vi "Agilent VNA Set Stimulus.vi"(7 "Agilent VNA":T4={"Model"="8753C", "Serial"="", "Firmware"="", "Learn String"=""}, 8 "error in (no error)":errorcluster, 9 "Channel":i8=1 min=1 max=99 step=1, 10 "Stimulus":T1={"Use Instrument Settings"=FALSE, "Blank Frequencies"=FALSE, "Sweep Type"=enum."Linear", "Sweep"={"Fstart"=500.0, "Fstop"=1500.0, "Units"=enum."MHz", "Points"=201}, "Power (dBm)"=999.0, "IFBW (Hz)"=-1.0, "Sweep Time (s)"=-1.0, "Calibration"={"State"=FALSE, "String"=""}} {"Sweep Time (s)" format="%.3g"}, 11 "VISA Resource Name":refnum<visa-resource-name>) -> (0 "error out":errorcluster {"code" format="%.0x"}, 3 "dup VISA Resource Name":refnum<visa-resource-name>)   [LabVIEW 2011]
uses:
  TypeDefs/Agilent VNA Instrument Info.ctl
  tests/S Parameter/TypeDefs/SP Stimulus Parameters.ctl
  tests/S Parameter/TypeDefs/SP Frequency Units.ctl
  tests/S Parameter/TypeDefs/SP Calibration State.ctl
  TypeDefs/Agilent VNA Sweep Type.ctl
  TypeDefs/Agilent VNA Trigger Mode.ctl
panel:
  in  "Case Constant\n(See Context Help)":bool
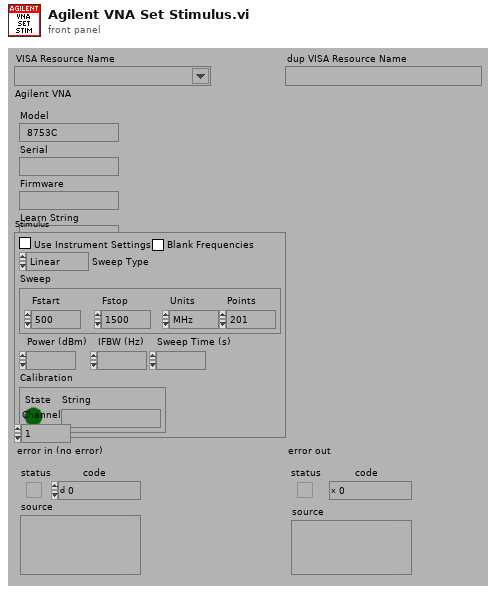
[diagram p1: front panel]
types:
  T1 = typedef "SP Stimulus Parameters.ctl" = cluster{"Use Instrument Settings":bool, "Blank Frequencies":bool, "Sweep Type":enum32{"Linear", "Logarithmic", "List", "Power", "CW"}, "Sweep":cluster{"Fstart":dbl, "Fstop":dbl, "Units":T2, "Points":i32}, "Power (dBm)":dbl, "IFBW (Hz)":dbl, "Sweep Time (s)":dbl, "Calibration":T3}
  T2 = typedef "SP Frequency Units.ctl" = enum16{"Hz", "kHz", "MHz", "GHz", "Points"}
  T3 = typedef "SP Calibration State.ctl" = cluster{"State":bool, "String":string}
  T4 = typedef "Agilent VNA Instrument Info.ctl" = cluster{"Model":string, "Serial":string, "Firmware":string, "Learn String":string}
  T5 = typedef "Agilent VNA Sweep Type.ctl" = enum32{"Linear Sweep", "Logarithmic Sweep", "Frequency List", "CW Time Sweep", "Power Sweep"}
  T6 = typedef "Agilent VNA Model.ctl" = enum16{"Not Supported", "8510X", "8719X", "8720X", "8722X", "8753X", "ENA", "PNA", "Field Fox"}
  T7 = typedef "Agilent VNA Trigger Mode.ctl" = enum16{"Continuous", "Hold", "Single"}
  T8 = enum32{"Linear", "Logarithmic", "List", "Power", "CW"}
  T9 = cluster{"Converted Frequency":dbl, "Converted Frequency":dbl}
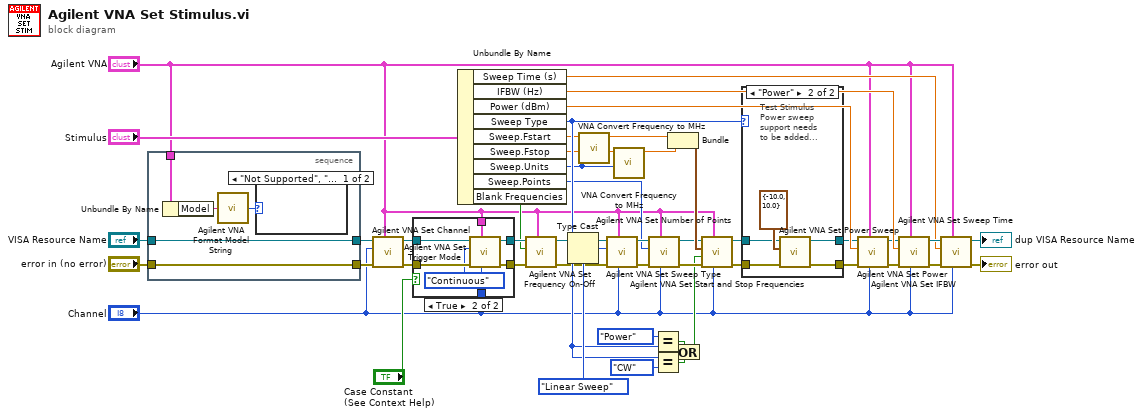
[diagram p0: block diagram]
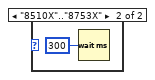
[diagram p3: hidden frame]
diagram:
  n1 = stacked-sequence {
    tunnel: "error in (no error)" -> [w52]
    tunnel: [w52] -> w34
    tunnel: "VISA Resource Name" -> [w51]
    tunnel: [w51] -> w32
    tunnel: "Agilent VNA" -> [w49]
    frame #0 {
      n2 = Unbundle By Name(w49) -> ("Model"=w48:string)
      n3 = call "Agilent VNA Format Model String.vi"("Model"=w48) -> ("Model"=w50:T6)
      n4 = case shown="\"Not Supported\", \"ENA\"..\"Field Fox\"" w50 {
        frame "Not Supported", "ENA".."Field Fox" {
        }
        frame "8510X".."8753X" {
          n5 = Wait (ms)(milliseconds to wait=u32 300) -> ()  [unwired: 1 out]
        }
      }
    }
  }
  n6 = call "Agilent VNA Set Channel.vi"("Agilent VNA"="Agilent VNA", "error in (no error)"=w34, "Channel"="Channel", "VISA Resource Name"=w32) -> ("error out"=w37:errorcluster, "dup VISA Resource Name"=w36:refnum<visa-resource-name>)  [unwired: 6 out]
  n7 = case shown="True" "Case Constant\n(See Context Help)" {
    tunnel: [w55 w59] -> w13
    tunnel: [w54 w60] -> w12
    tunnel: w37 -> [w55 w62]
    tunnel: w36 -> [w54 w61]
    tunnel: "Agilent VNA" -> [_ w57]
    tunnel: "Channel" -> [_ w56]
    frame False {
    }
    frame True {
      n8 = call "Agilent VNA Set Trigger Mode.vi"("Channel"=w56, "Agilent VNA"=w57, "error in (no error)"=w62, "Trigger Mode"=Agilent_VNA_Trigger_Mode."Continuous", "VISA Resource Name"=w61) -> ("error out"=w59:errorcluster, "dup VISA Resource Name"=w60:refnum<visa-resource-name>)  [unwired: 5 out]
    }
  }
  n9 = Unbundle By Name("Stimulus") -> ("Sweep Time (s)"=w40:dbl, "IFBW (Hz)"=w45:dbl, "Power (dBm)"=w46:dbl, "Sweep Type"=w16:T8, "Sweep.Fstart"=w6:dbl, "Sweep.Fstop"=w5:dbl, "Sweep.Units"=w4:T2, "Sweep.Points"=w7:i32, "Blank Frequencies"=w9:bool)
  n10 = call "Agilent VNA Set Frequency On-Off.vi"("Agilent VNA"="Agilent VNA", "error in (no error)"=w13, "Blank Frequencies (F)"=w9, "VISA Resource Name"=w12) -> ("error out"=w10:errorcluster, "dup VISA Resource Name"=w11:refnum<visa-resource-name>)  [unwired: 6 out]
  n11 = Type Cast(type=Agilent_VNA_Sweep_Type."Linear Sweep" ("Sweep Type"), x=w16) -> (*(type *) &x=w28:T5)
  n12 = call "VNA Convert Frequency to MHz.vi"("Units"=w4, "Frequency"=w6) -> ("Converted Frequency"=w3:dbl)  [unwired: 9 out]
  n13 = call "Agilent VNA Set Sweep Type.vi"("Channel"="Channel", "Agilent VNA"="Agilent VNA", "error in (no error)"=w10, "Sweep Type"=w28, "VISA Resource Name"=w11) -> ("error out"=w23:errorcluster, "dup VISA Resource Name"=w24:refnum<visa-resource-name>)  [unwired: 5 out]
  n14 = call "VNA Convert Frequency to MHz.vi"("Units"=w4, "Frequency"=w5) -> ("Converted Frequency"=w2:dbl)  [unwired: 9 out]
  n15 = call "Agilent VNA Set Number of Points.vi"("Channel"="Channel", "Agilent VNA"="Agilent VNA", "error in (no error)"=w23, "Number Points"=w7, "VISA Resource Name"=w24) -> ("error out"=w25:errorcluster, "dup VISA Resource Name"=w26:refnum<visa-resource-name>)  [unwired: 5 out]
  n16 = Equal?(x=enum32{"Linear", "Log", "List", "Power", "CW"}."Power" ("Sweep Type"), y=w16) -> (x = y?=w20:bool)
  n17 = Equal?(x=w16, y=enum32{"Linear", "Log", "List", "Power", "CW"}."CW" ("Sweep Type")) -> (x = y?=w19:bool)
  n18 = Bundle("Converted Frequency"=w3, "Converted Frequency"=w2) -> (w27:T9)  [unwired: 1 out]
  n19 = Or(x=w20, y=w19) -> (x .or. y?=w15:bool)
  n20 = call "Agilent VNA Set Start and Stop Frequencies.vi"("Channel"="Channel", "Agilent VNA"="Agilent VNA", "error in (no error)"=w25, "CW? (f)"=w15, "Start/Stop Freqs, MHz"=w27, "VISA Resource Name"=w26) -> ("error out"=w22:errorcluster, "dup VISA Resource Name"=w21:refnum<visa-resource-name>)  [unwired: 4 out]
  n21 = case shown="\"Power\"" w16 {
    tunnel: w22 -> [w64 w66]
    tunnel: w21 -> [w63 w65]
    tunnel: [w63 w68] -> w44
    tunnel: [w64 w67] -> w43
    frame "Linear", "Logarithmic", "CW", Default {
    }
    frame "Power" {
      # "Test Stimulus\nPower sweep\nsupport needs\nto be added..."
      n22 = call "Agilent VNA Set Power Sweep.vi"("error in (no error)"=w66, "Start/Stop Power, dBm"=cluster{"Pstart":dbl, "Pstop":dbl} {"Pstart"=-10.0, "Pstop"=10.0}, "VISA Resource Name"=w65) -> ("error out"=w67:errorcluster, "dup VISA Resource Name"=w68:refnum<visa-resource-name>)  [unwired: 7 out]
    }
  }
  n23 = call "Agilent VNA Set Power.vi"("Channel"="Channel", "Agilent VNA"="Agilent VNA", "error in (no error)"=w43, "Source Power, dBm (0.0)"=w46, "VISA Resource Name"=w44) -> ("error out"=w39:errorcluster, "dup VISA Resource Name"=w38:refnum<visa-resource-name>)  [unwired: 5 out]
  n24 = call "Agilent VNA Set IFBW.vi"("Channel"="Channel", "Agilent VNA"="Agilent VNA", "error in (no error)"=w39, "IFBW, Hz (3000)"=w45, "VISA Resource Name"=w38) -> ("error out"=w42:errorcluster, "dup VISA Resource Name"=w41:refnum<visa-resource-name>)  [unwired: 5 out]
  n25 = call "Agilent VNA Set Sweep Time.vi"("Channel"="Channel", "Agilent VNA"="Agilent VNA", "error in (no error)"=w42, "Sweep Time, s (-1: Auto)"=w40, "VISA Resource Name"=w41) -> ("error out"=→"error out":errorcluster, "dup VISA Resource Name"=→"dup VISA Resource Name":refnum<visa-resource-name>)  [unwired: 5 out]
